vi "Host_side_DAQ_data.vi"() -> ()   [LabVIEW 2017]
uses:
  <vilib>/Waveform/WDTOps.llb/WDT Append Waveforms DBL.vi
panel:
  in  "stop":bool
  out "Waveform Chart":waveform(dbl)(graph)
  in  "Recording Data":bool
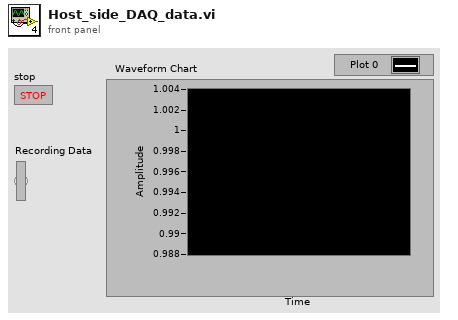
[diagram p1: front panel]
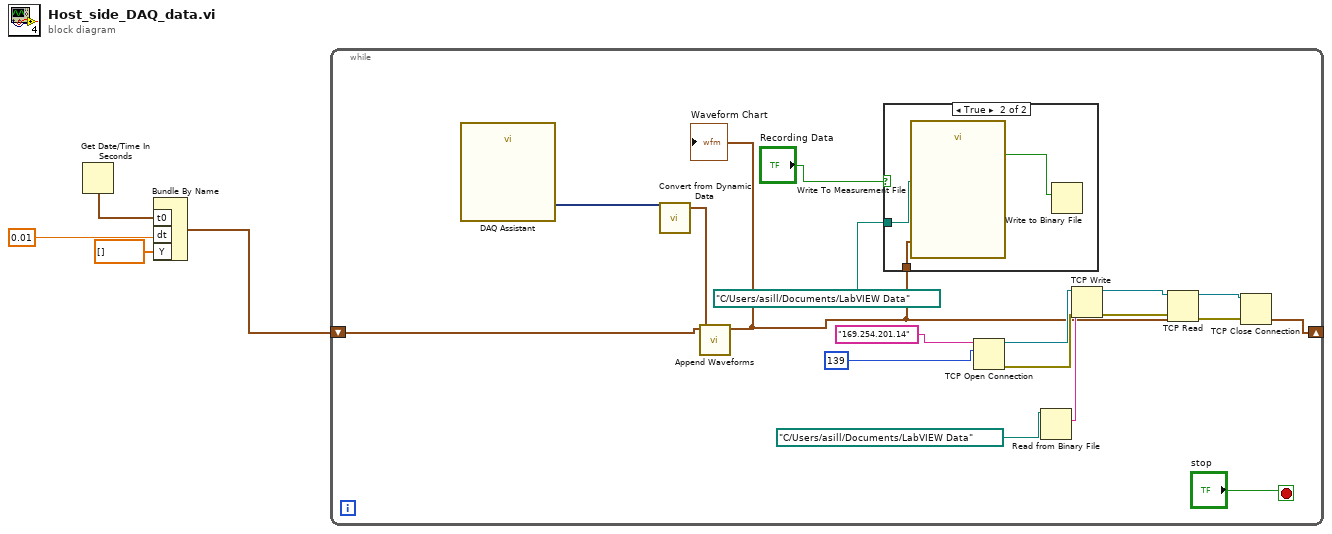
[diagram p0: block diagram]
diagram:
  n1 = Get Date/Time In Seconds() -> (seconds since 1Jan1904=w2:timestamp)
  n2 = Bundle By Name("t0"=w2, "dt"=0.01, "Y"=dbl[] []) -> (w3:waveform(dbl))  [unwired: 1 in]
  n3 = while {
    shift-right: [w8] -> _
    shift-left: w3 -> [w20]
    stop <- "stop" stop-if-true
    n4 = call "DAQ Assistant"() -> ("data"=w19:dynamicdata)  [unwired: 16 in, 3 out]
    n5 = call "Convert from Dynamic Data"("Dynamic Data Type"=w19) -> ("Waveform"=w18:waveform(dbl))  [unwired: 3 in]
    n6 = call-poly <vilib>:"Append Waveforms.vi"("waveform B"=w18, "waveform A"=w20) -> ("waveform out"=w8:waveform(dbl))  [unwired: 8 in, 1 out]
    "Waveform Chart" <- w8
    n7 = case shown="True" "Recording Data" {
      tunnel: w8 -> [_ w24]
      tunnel: path "C:/Users/asill/Documents/LabVIEW Data" -> [_ w22]
      frame False {
      }
      frame True {
        n8 = call "Write To Measurement File"("Signals"=w24, "Filename"=w22) -> ("Saving Data"=w23:bool)  [unwired: 15 in, 2 out]
        n9 = Write to Binary File(data=w23) -> ()  [unwired: 5 in, 3 out]
      }
    }
    n10 = TCP Open Connection(address="169.254.201.14", remote port or service name=139) -> (connection ID=w16:refnum<k5>, error out=w13:errorcluster)  [unwired: 3 in]
    n11 = Read from Binary File(11:path "C:/Users/asill/Documents/LabVIEW Data") -> (2:w9:string)  [unwired: 5 in, 3 out]
    n12 = TCP Write(connection ID=w16, data in=w9, error in (no error)=w13) -> (connection ID out=w15:refnum<k5>, error out=w12:errorcluster)  [unwired: 1 in, 1 out]
    n13 = TCP Read(connection ID=w15, error in (no error)=w12) -> (connection ID out=w14:refnum<k5>, error out=w11:errorcluster)  [unwired: 3 in, 1 out]
    n14 = TCP Close Connection(connection ID=w14, error in (no error)=w11) -> ()  [unwired: 1 in, 2 out]
  }
